vi "SendMultipleMessages.vi"(6 "timeout in ms (-1)":i32=-1, 8 "error in":errorcluster, 9 "message data []":variant[](array[variant]), 10 "message names []":string[](array[string]), 11 "message ref in":refnum<class "CLM_LocalMessage_Queue.lvclass">) -> (0 "error out":errorcluster, 3 "message ref out":refnum<class "CLM_LocalMessage_Queue.lvclass">, 4 "timed out?":bool)   [LabVIEW 2013, in "CLM_LocalMessage_Queue.lvclass"]
uses:
  CLM_LocalMessage_Queue.lvclass
  CLM_LocalMessage_Queue.lvclass/CLM_LocalMessage_Queue.ctl
  SendQueueMessage.vi
  SendQueueMessage_Cluster.vi
  LocalMessage/BundleMessageCluster.vi
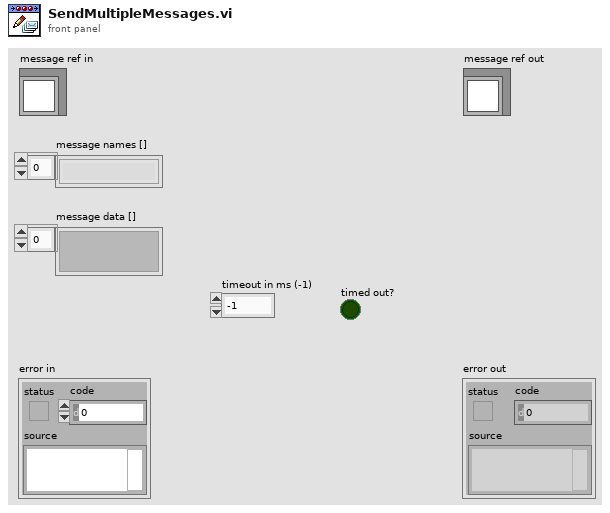
[diagram p1: front panel]
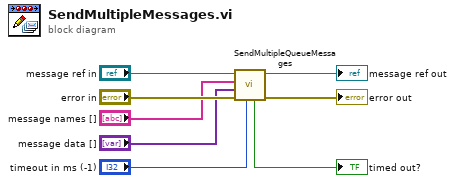
[diagram p0: block diagram]
diagram:
  n1 = call "SendMultipleQueueMessages.vi"("timeout in ms (-1)"="timeout in ms (-1)", "error in"="error in", "message data []"="message data []", "message names []"="message names []", "message ref in"="message ref in") -> ("error out"=→"error out":errorcluster, "message ref out"=→"message ref out":refnum<class "CLM_LocalMessage_Queue.lvclass">, "timed out?"=→"timed out?":bool)  [unwired: 4 in]
